vi "Open SenseHat.Display.vi"(8 "error in (no error)":errorcluster, 11 "LINX Resource":T1) -> (0 "error out":errorcluster, 3 "senseHatDisplay out":refnum<class "RPI.SenseHat.Display.lvclass">)   [LabVIEW 2020, in "RPI.SenseHat.Display.lvlib" / "RPI.SenseHat.Display.lvclass"]
doc: "Instantiates a RPI.SenseHat.Display object.\n\nNote: opens the I2C communication."
uses:
  RPI.SenseHat.Display.lvclass
  <vilib>/MakerHub/LINX/Private/Type Defs/LINX Ref.ctl
  <vilib>/MakerHub/LINX/Private/Type Defs/Platform.ctl
  <vilib>/MakerHub/LINX/Private/Type Defs/Interface.ctl
  <vilib>/MakerHub/LINX/Private/Device/Type Defs/LINX Device Config.ctl
  <vilib>/MakerHub/LINX/Private/Device/Type Defs/TCP Config.ctl
  <vilib>/MakerHub/LINX/Private/Device/Type Defs/Channels.ctl
  TypeDefs/Display Direction.ctl
  RPI.SenseHat.Display.lvclass/RPI.SenseHat.Display.ctl
  RPI/Classes/mainI2CDevice/mainI2CDevice.lvclass
  RPI.SenseHat.Display.lvlib
  Image/Image.lvclass
  <vilib>/MakerHub/LINX/LMH-LINX.lvlib
  <vilib>/MakerHub/LINX/Private/Device/Device.lvlib
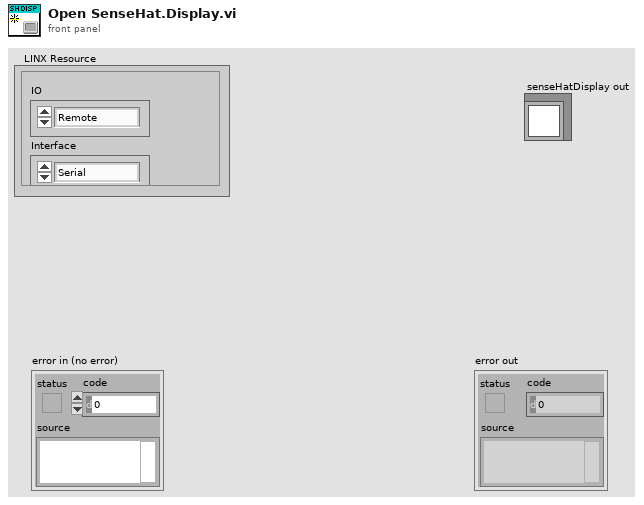
[diagram p1: front panel]
types:
  T1 = typedef "LMH-LINX.lvlib/LINX Ref.ctl" = cluster{"IO":T2, "Interface":T3, "LINX Device Config":T4}
  T2 = typedef "LMH-LINX.lvlib/Platform.ctl" = enum16{"Remote", "Local"}
  T3 = typedef "LMH-LINX.lvlib/Interface.ctl" = enum16{"Serial", "TCP"}
  T4 = typedef "LMH-LINX.lvlib/Device.lvlib/LINX Device Config.ctl" = cluster{"Interface":T3, "COM Port":refnum<visa-resource-name>, "TCP Configuration":T5, "Device Family":u8, "Device ID":u8, "Device Name":string, "TCP Ref":refnum<k5>, "Channels":T6}
  T5 = typedef "LMH-LINX.lvlib/Device.lvlib/TCP Config.ctl" = cluster{"IP Address":string, "Port":u16}
  T6 = typedef "LMH-LINX.lvlib/Channels.ctl" = cluster{"DI":u8[], "DO":u8[], "AI":u8[], "AO":u8[], "PWM":u8[], "QE":u8[], "UART":u8[], "I2C 2":u8[], "SPI":u8[], "CAN":u8[], "Servo":u8[], "AI Ref (V)":dbl, "AI Resolution (Bits)":u8, "AO Ref (V)":dbl, "AO Resolution (Bits)":u8}
  T7 = typedef "RPI.SenseHat.Display.lvlib/Display Direction.ctl" = enum16{"deg0", "deg90", "deg180", "deg270"}
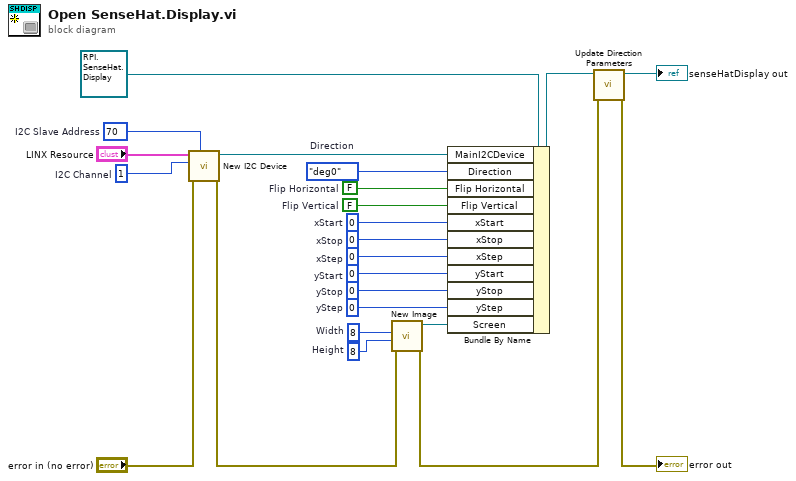
[diagram p0: block diagram]
diagram:
  w4 = 8  # Width
  w5 = 8  # Height
  w9 = 0  # yStep
  w10 = 0  # yStop
  w11 = 0  # yStart
  w12 = 0  # xStep
  w13 = 0  # xStop
  w14 = 0  # xStart
  w15 = FALSE  # Flip Vertical
  w16 = FALSE  # Flip Horizontal
  w17 = Display_Direction."deg0"  # Direction
  w21 = u8 1  # I2C Channel
  w8 = u8 70  # I2C Slave Address
  n1 = call "New I2C Device.vi"("I2C Slave Address"=w8, "error in (no error)"="error in (no error)", "I2C Channel"=w21, "object in"="LINX Resource") -> ("error out"=w6:errorcluster, "mainI2CDevice out"=w18:refnum<class "mainI2CDevice.lvclass">)  [unwired: 6 in]
  n2 = call "New Image.vi"("error in (no error)"=w6, "Height"=w5, "Width"=w4) -> ("error out"=w2:errorcluster, "Image out"=w7:refnum<class "Image.lvclass">)  [unwired: 7 in]
  n3 = Bundle By Name(cluster=refnum<class "RPI.SenseHat.Display.lvclass"> refnum ("senseHatDisplay in"), "MainI2CDevice"=w18, "Direction"=w17, "Flip Horizontal"=w16, "Flip Vertical"=w15, "xStart"=w14, "xStop"=w13, "xStep"=w12, "yStart"=w11, "yStop"=w10, "yStep"=w9, "Screen"=w7) -> (w19:refnum<class "RPI.SenseHat.Display.lvclass">)
  n4 = call "Update Direction Parameters.vi"("error in (no error)"=w2, "senseHatDisplay in"=w19) -> ("error out"=→"error out":errorcluster, "senseHatDisplay out"=→"senseHatDisplay out":refnum<class "RPI.SenseHat.Display.lvclass">)  [unwired: 8 in]
